vi "Read String.vi"(8 "error in":errorcluster, 10 "Name":string, 11 "Handle In":i32) -> (0 "error out":errorcluster, 2 "String":string, 3 "Handle Out":i32, 4 "Error Frame":i32)   [LabVIEW 2024]
panel:
  out "String Length":i32
  out "Values Out":dbl[](array[numeric]) format="%.2f"
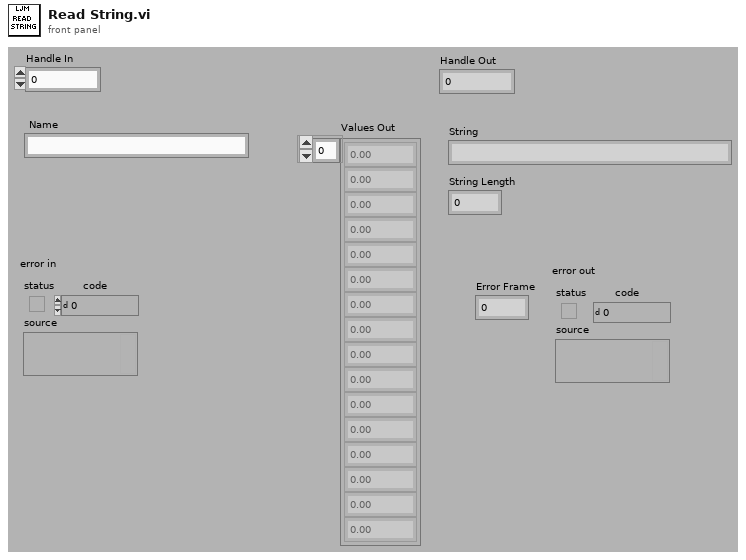
[diagram p1: front panel]
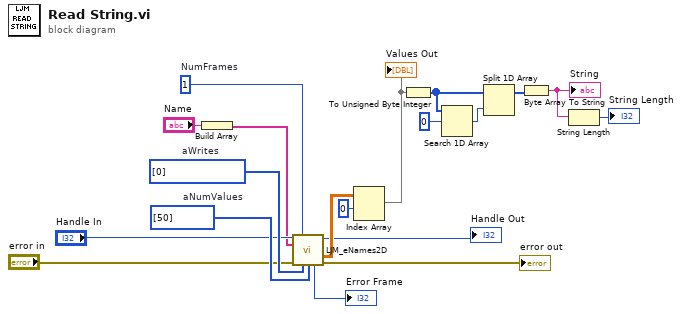
[diagram p0: block diagram]
diagram:
  w14 = i32[] [50]  # aNumValues
  w15 = i32[] [0] items=["Read", "Write"]  # aWrites
  w16 = 1  # NumFrames
  n1 = Build Array("Name") -> (w1:string[])
  n2 = call "LJM_eNames2D.vi"("Handle In"="Handle In", "NumFrames (Auto-Detect)"=w16, "aNames"=w1, "error in"="error in", "aWrites"=w15, "aNumValues"=w14) -> ("Handle Out"=→"Handle Out":i32, "aValuesOut"=w13:dbl[][], "ErrorAddress"=→"Error Frame":i32, "error out"=→"error out":errorcluster)  [unwired: 6 in]
  n3 = Index Array(array=w13, index (row)=0 ("Index (row)")) -> (element=w11:dbl[])  [unwired: 1 in]
  "Values Out" <- w11
  n4 = To Unsigned Byte Integer(number=w11) -> (unsigned 8bit integer=w9:u8[])
  n5 = Search 1D Array(1D array=w9, element=u8 0) -> (index of element=w8:i32)  [unwired: 1 in]
  n6 = Split 1D Array(array=w9, index=w8) -> (first subarray=w7:u8[])  [unwired: 1 out]
  n7 = Byte Array To String(unsigned byte array=w7) -> (string=w18:string)
  "String" <- w18
  n8 = String Length(string=w18) -> (length=→"String Length":i32)
